vi "ASE_MPC_Experiment_template.vi"() -> ()   [LabVIEW 2018]
uses:
  <vilib>/Simulation/Scripting/Companion Diagram/SimConfigNode/SimParams.ctl
  <vilib>/Simulation/Scripting/Companion Diagram/SimConfigNode/_simSolvers.ctl
  <vilib>/Simulation/Implementation/Shared/SIMSCR Execution Mode.ctl
  <vilib>/Platform/TimedLoop/XDataNode/timing_clust.ctl
  <vilib>/Platform/TimedLoop/XDataNode/nitl_modes.ctl
  <vilib>/Platform/TimedLoop/XDataNode/wakeup.ctl
  <vilib>/Simulation/Param Hierarchy/Typedefs/SIMPH Param Control Actions.ctl
  <vilib>/Simulation/Implementation/Shared/SIM limit type.ctl
  <vilib>/Simulation/Scripting/Editor Utilities/SIM subVI tag data.ctl
  <vilib>/Simulation/Scripting/Editor Utilities/SIM subVI execution type.ctl
  <vilib>/Simulation/Implementation/Shared/NILVSim_ParamChanged.vi
  <vilib>/Simulation/Implementation/Shared/NILVSim_FinishedLate.vi
  <vilib>/Simulation/Implementation/Shared/NILVSIM_BeginStep.vi
  <vilib>/Simulation/Utility/Implementation/SIM Halt.vi
  <vilib>/Simulation/DataSources/Implementation/NILVSim Signal Generator.llb/SIM Signal Generator (scalar).vi
  <vilib>/Simulation/Nonlinear/Implementation/NILVSim Saturation.llb/SIM Saturation (scalar).vi
  <vilib>/Simulation/ContinuousLinear/Implementation/NILVSim Transfer Function.llb/SIM Transfer Function Distributor (SISO).vi
  <vilib>/Simulation/SignalArithmetic/Implementation/NILVSim Gain.llb/SIM Gain (scalar).vi
  <vilib>/Simulation/ContinuousLinear/Implementation/NILVSim Integrator new.llb/SIM Integrator distributor (scalar).vi
  <vilib>/Simulation/ContinuousLinear/Implementation/NILVSim Transfer Function.llb/SIM Transfer Function Collector (SISO).vi
  <vilib>/Simulation/Nonlinear/Implementation/NILVSim RateLimiter.llb/SIM RateLimiter (scalar).vi
  <vilib>/Simulation/Implementation/Shared/SIM Fire Discrete SubVI.vi
  <vilib>/Simulation/ContinuousLinear/Implementation/NILVSim Integrator new.llb/SIM Integrator collector (scalar).vi
  <vilib>/Simulation/Nonlinear/Implementation/NILVSim Saturation.llb/SIM Saturation (vector).vi
  <vilib>/Simulation/SignalArithmetic/Implementation/NILVSim Gain.llb/SIM Gain (vector).vi
  <vilib>/Simulation/Implementation/Shared/NILVSim_Manager.vi
  <vilib>/Utility/error.llb/Clear Errors.vi
  <vilib>/Simulation/Implementation/Shared/NILVSim_FinalizeModel.vi
  <vilib>/Simulation/Implementation/Shared/SIM Fire Discrete SubVI (Core).vi
  <vilib>/imath/engines/lvmath/Plug In/Control Design/BuiltInFunctions/ss/NIMS_CD_ss(A,B,C,D).vi
  <vilib>/imath/engines/lvmath/Plug In/Control Design/BuiltInFunctions/c_to_d/NIMS_CD_c_to_d(SS,TS,STR,DBL).vi
  <vilib>/imath/engines/lvmath2/RunTimeEngine/NodeEndStatement/NIMS_NodeEndStatement_Output.vi
  <instcachedir>/0/NIMS_NodeEndStatement_Output_53EC0D466D134D7ABD903AC30B43404B.lvgen/NIMS_NodeEndStatement_Output_53EC0D466D134D7ABD903AC30B43404B_011.vi
  <vilib>/imath/engines/lvmath2/RunTimeEngine/ErrorHandling/NIMS_Finalize Error.vi
  <vilib>/addons/Control Design/_Model Construction/Model Information.llb/Model Information SubVIs/cd_Get Matrices From SS Model.vi
  <vilib>/imath/engines/lvmath2/RunTimeEngine/IndexRead/NIMS V(R2).vi
  <instcachedir>/0/NIMS V(R2)_C76619605A0E4E9F8B2FA9389712AC47.lvgen/NIMS V(R2)_C76619605A0E4E9F8B2FA9389712AC47_000.vi
  <vilib>/imath/engines/lvmath2/RunTimeEngine/BuiltInFunctions/diag/NIMS_diag.vi
  <instcachedir>/0/NIMS_diag_A176D428AACC4FD18ED77B06CA0A1FE1.lvgen/NIMS_diag_A176D428AACC4FD18ED77B06CA0A1FE1_003.vi
  <vilib>/imathl/engines/lvmath/Functions/Error Handling/Create Error.vi
  <vilib>/imath/engines/lvmath2/RunTimeEngine/IndexRead/NIMS V(S).vi
  <instcachedir>/0/NIMS V(S)_0488751826AF41519A22953C041130DC.lvgen/NIMS V(S)_0488751826AF41519A22953C041130DC_000.vi
  <vilib>/imath/engines/lvmath2/RunTimeEngine/ArithmeticOperatorToken/NIMS_ArithmeticOperator_multmx.vi
  <instcachedir>/0/NIMS_ArithmeticOperator_multmx_622CA76F9646436AB036D42A9A1CE0E6.lvgen/NIMS_ArithmeticOperator_multmx_622CA76F9646436AB036D42A9A1CE0E6_004.vi
  <vilib>/imath/engines/lvmath2/RunTimeEngine/ArithmeticOperatorToken/NIMS_ArithmeticOperator_plus.vi
  <instcachedir>/0/NIMS_ArithmeticOperator_plus_DE670E32103C4C10ADF2A97367172B30.lvgen/NIMS_ArithmeticOperator_plus_DE670E32103C4C10ADF2A97367172B30_003.vi
  <vilib>/imath/engines/lvmath2/RunTimeEngine/ErrorHandling/NIMS_Create Error From Enums.vi
  <vilib>/imath/engines/lvmath2/RunTimeEngine/IndexReplace/NIMS M(S,S)=S.vi
  <instcachedir>/0/NIMS M(S,S)=S_5DAF17B45D8A4C8588C7CF468644990A.lvgen/NIMS M(S,S)=S_5DAF17B45D8A4C8588C7CF468644990A_002.vi
  <vilib>/imath/engines/lvmath2/RunTimeEngine/BuiltInFunctions/eye/NIMS_M=eye(I32, I32).vi
  <vilib>/imath/engines/lvmath2/RunTimeEngine/IndexReplace/NIMS M(R2,$)=M.vi
  <instcachedir>/0/NIMS M(R2,$)=M_E62C22E4B8174738B7B297CD2875EB66.lvgen/NIMS M(R2,$)=M_E62C22E4B8174738B7B297CD2875EB66_002.vi
  <vilib>/imath/engines/lvmath2/RunTimeEngine/RangeToken/NIMS_Range_R2 - Integer.vi
  <instcachedir>/0/NIMS_Range_R2 - Integer_E35B921DECF84AADB7325A02D418BFCC.lvgen/NIMS_Range_R2 - Integer_E35B921DECF84AADB7325A02D418BFCC_001.vi
  <vilib>/imath/engines/lvmath2/RunTimeEngine/CommandStatement/MC_CommandStatement_break.vi
  <vilib>/imath/engines/lvmath2/RunTimeEngine/ArithmeticOperatorToken/NIMS_ArithmeticOperator_powermx(M,M).vi
  <instcachedir>/0/NIMS_ArithmeticOperator_multmx_622CA76F9646436AB036D42A9A1CE0E6.lvgen/NIMS_ArithmeticOperator_multmx_622CA76F9646436AB036D42A9A1CE0E6_006.vi
  <vilib>/imath/engines/lvmath2/RunTimeEngine/MatrixToken/NIMS_MatrixToken_M_M.vi
  <instcachedir>/0/NIMS_MatrixToken_M_M_C5809CB3B49B4BB3BF486E1039DE826B.lvgen/NIMS_MatrixToken_M_M_C5809CB3B49B4BB3BF486E1039DE826B_003.vi
  <instcachedir>/0/NIMS_ArithmeticOperator_multmx_622CA76F9646436AB036D42A9A1CE0E6.lvgen/NIMS_ArithmeticOperator_multmx_622CA76F9646436AB036D42A9A1CE0E6_007.vi
  <vilib>/imath/engines/lvmath2/RunTimeEngine/IndexReplace/NIMS M(R2,R2)=M.vi
  <instcachedir>/0/NIMS M(R2,R2)=M_33171D760B764D5F81A0D4DA8D20878D.lvgen/NIMS M(R2,R2)=M_33171D760B764D5F81A0D4DA8D20878D_000.vi
  <instcachedir>/0/NIMS M(S,S)=S_5DAF17B45D8A4C8588C7CF468644990A.lvgen/NIMS M(S,S)=S_5DAF17B45D8A4C8588C7CF468644990A_000.vi
  <instcachedir>/0/NIMS_ArithmeticOperator_multmx_622CA76F9646436AB036D42A9A1CE0E6.lvgen/NIMS_ArithmeticOperator_multmx_622CA76F9646436AB036D42A9A1CE0E6_003.vi
  <vilib>/imath/engines/lvmath2/RunTimeEngine/RowToken/NIMS_RowToken_M_M.vi
  <instcachedir>/0/NIMS_RowToken_M_M_9381229BAB584C0281F245468A1A9A6C.lvgen/NIMS_RowToken_M_M_9381229BAB584C0281F245468A1A9A6C_003.vi
  <instcachedir>/0/NIMS_ArithmeticOperator_plus_DE670E32103C4C10ADF2A97367172B30.lvgen/NIMS_ArithmeticOperator_plus_DE670E32103C4C10ADF2A97367172B30_011.vi
  <instcachedir>/0/NIMS_NodeEndStatement_Output_53EC0D466D134D7ABD903AC30B43404B.lvgen/NIMS_NodeEndStatement_Output_53EC0D466D134D7ABD903AC30B43404B_002.vi
  <instcachedir>/0/NIMS_NodeEndStatement_Output_53EC0D466D134D7ABD903AC30B43404B.lvgen/NIMS_NodeEndStatement_Output_53EC0D466D134D7ABD903AC30B43404B_003.vi
  <instcachedir>/0/NIMS_NodeEndStatement_Output_53EC0D466D134D7ABD903AC30B43404B.lvgen/NIMS_NodeEndStatement_Output_53EC0D466D134D7ABD903AC30B43404B_012.vi
  <vilib>/FPGAPlugInAG/cRIO-9068/niLvFpga_Open_cRIO-9068.vi
  <vilib>/rvi/interface/common/dynamic/niFpgaDynamicAddResources.vi
  <vilib>/Simulation/Implementation/Shared/SIM Unbundle Sim Info.vi
  <vilib>/Simulation/Implementation/Shared/SIMSH Read Queue.vi
  <vilib>/Simulation/Implementation/Shared/NILVSim_Initialize.vi
  <vilib>/Utility/error.llb/Error Cluster From Error Code.vi
  <vilib>/rvi/errors/niLvFpgaAdjustHostInterfaceError.vi
  <vilib>/Simulation/Utility/Implementation/NILVSim Get Time and IsAcceptedStep.vi
  <vilib>/imath/engines/lvmath2/RunTimeEngine/ArithmeticOperatorToken/NIMS_ArithmeticOperator_multmx(M,CV).vi
  <instcachedir>/0/NIMS_ArithmeticOperator_multmx(M,CV)_2F1CD6A2FE4F4213A4AD1C901C2750F5.lvgen/NIMS_ArithmeticOperator_multmx(M,CV)_2F1CD6A2FE4F4213A4AD1C901C2750F5_002.vi
  <vilib>/imath/engines/lvmath2/RunTimeSupport/NIMS_Complex To Real.vi
  <instcachedir>/0/NIMS_Complex To Real_DC07FF5F56D84FD694198341FF08C5E7.lvgen/NIMS_Complex To Real_DC07FF5F56D84FD694198341FF08C5E7_000.vi
  <vilib>/imath/engines/lvmath2/RunTimeSupport/NIMS_Get Any Vector_w Error - Matrix.vi
  <instcachedir>/0/NIMS_Get Any Vector_w Error - Matrix_1B26302039EC43C7B9FA287B1E12D88C.lvgen/NIMS_Get Any Vector_w Error - Matrix_1B26302039EC43C7B9FA287B1E12D88C_001.vi
  <vilib>/imath/engines/lvmath2/RunTimeEngine/BuiltInFunctions/fmin_qp/NIMS_fmin_qp.vi
  <instcachedir>/0/NIMS_NodeEndStatement_Output_53EC0D466D134D7ABD903AC30B43404B.lvgen/NIMS_NodeEndStatement_Output_53EC0D466D134D7ABD903AC30B43404B_001.vi
  <vilib>/Simulation/Implementation/Shared/NILVSim_GetModelError.vi
  <vilib>/Simulation/Implementation/Shared/SIM Bundle Sim Info.vi
  <vilib>/FPGAPlugInAG/Dynamic/niLvFpga_Close_Dynamic.vi
  <vilib>/Simulation/Scripting/Companion Diagram/SimConfigNode/SimDog.xnode
  <vilib>/rvi/interface/nirviOpenFPGA/nirviOpenFPGA.xnode
  FPGA Bitfiles/MPCASE_FPGATarget_FPGAQ1MODULE_QZL3H99B2Ro.lvbitx
  FPGA_Q1_MODULE.vi
  <vilib>/Quanser/Rapid Control Prototyping Toolkit/discrete/_TypeSpecific/CL Bias Removal (Scalar).vi
  <vilib>/Quanser/Rapid Control Prototyping Toolkit/discrete/CL Bias Removal.vi
  <vilib>/Platform/TimedLoop/XDataNode/XDataNode.xnode
  <vilib>/rvi/interface/nirviReadWriteControl/nirviReadWriteControl.xnode
  <vilib>/Simulation/Implementation/XNodeFramework/SimXNode/SimX.xnode
  <vilib>/rvi/interface/nirviCloseFPGA/nirviCloseFPGA.xnode
  <vilib>/Simulation/ContinuousLinear/Implementation/NILVSim Transfer Function.llb/SIM Transfer Function (SISO).vi
  <vilib>/Simulation/ContinuousLinear/Implementation/NILVSim Integrator new.llb/SIM Integrator (scalar).vi
  <vilib>/rvi/interface/Simulation/niFpgaSimulationCallBeginRW.vi
  <vilib>/addons/Control Design/_Model Construction/NI_LinSys_Model Information.lvlib
  NiFpgaLv.dll
  <vilib>/Platform/TimedLoop/XDataNode/XDNodeRunTimeDep.lvlib
  <vilib>/Simulation/Implementation/Shared/NI_SIM_Implementation.lvlib
panel:
  out "A":dbl[][](array[numeric])
  in  "weight O4":dbl
  in  "weight O3":dbl
  in  "weight I1":dbl
  in  "weight O2":dbl
  in  "weight O1":dbl
  in  "Control Horizon (Nc)":u64 step=1
  in  "Prediction Horizon (Np)":u64 step=1
  in  "Enable motor":bool
  in  "Setpoint Command 2":T1={"Amplitude (m)"=0.01, "Frequency (Hz)"=0.3} caption="Road (Bottom Plate)\nAmplitude Command (m)" {"Frequency (Hz)" min=0.0 max=0.5 step=0.009999999776482582 format="%_3f"; "Amplitude (m)" min=-10.0 max=10.0 step=0.5 format="%_3f"}
  out "Active Suspension Motor Voltage (V)":dbl(graph)
  in  "Enable active suspension":bool
  out "Zr(m), Zs(m), Zus(m) 2":T2(graph)={"output"=0.0096065956, "Result"=0.0090666584, "output"=0.0091514816}
  out "Accelerometer Signal":dbl(graph)
  in  "Halt?":bool
  # "Active Suspension MPC"
  # "MPC parameters"
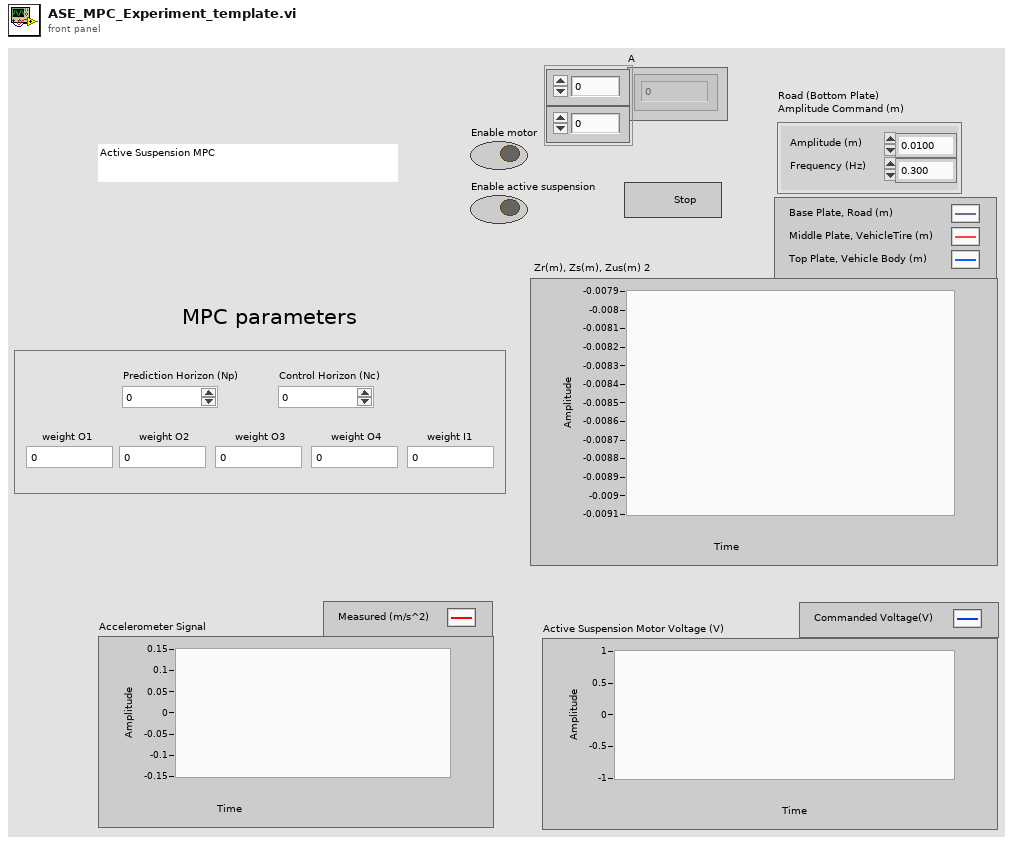
[diagram p1: front panel]
types:
  T1 = cluster{"Amplitude (m)":dbl, "Frequency (Hz)":dbl}
  T2 = cluster{"output":dbl, "Result":dbl, "output":dbl}
  T3 = typedef "SIMSCR Execution Mode.ctl" = enum16{"Simulate to Completion", "Single Time-Step Simulation (Fixed Step Only)"}
  T4 = typedef "XDNodeRunTimeDep.lvlib/timing_clust.ctl" = cluster{"Expected End [f-1]":u64, "Actual End [f-1]":u64, "Finished Late? [f-1]":bool, "Expected End [i-1]":u64, "Actual End [i-1]":u64, "Finished Late? [i-1]":bool, "Expected Start [i]":u64, "Actual Start [i]":u64, "Expected Start [f]":u64, "Actual Start [f]":u64, "Source Name":string, "Structure Name":string, "Period":i64, "Deadline":i64, "Offset":i64, "Start":i64, "Priority":i32, "Timeout":i32, "Mode":T5, "Wakeup Reason":T6, "Error":errorcluster, "Source Type":string, "Secondary Source Type":string, "Global End Time":u64, "Global Start Time":u64, "Frame Duration":u64, "Iteration Duration":u64, "Assigned CPU":i32, "I/O Scan Engine Mode":u32}
  T5 = typedef "XDNodeRunTimeDep.lvlib/nitl_modes.ctl" = enum32{"No Change", "Process missed periods, maintain original phase", "Discard missed periods, maintain original phase", "Process missed periods, ignore original phase", "Discard missed periods, ignore original phase"}
  T6 = typedef "XDNodeRunTimeDep.lvlib/wakeup.ctl" = enum32{"Normal", "Aborted", "Asynchronous wakeup", "Timing source error", "Timed loop error", "Timeout"}
  T7 = typedef "SIMPH Param Control Actions.ctl" = enum16{"get params", "set params"}
  T8 = typedef "SIM subVI tag data.ctl" = cluster{"period":dbl, "skew":dbl, "Simulation execution type":T9}
  T9 = typedef "SIM subVI execution type.ctl" = enum16{"Function call", "Discrete", "Continuous", "Initialization only", "Final step only"}
  T10 = typedef "SIM limit type.ctl" = enum16{"upper", "lower", "both", "none"}
  T11 = cluster{"SIMSH Sim Time":dbl, "CL Enabled Moving Average (Scalar)":cluster{"output":dbl}, "CL Enabled Moving Average (Scalar) - SIMSH":cluster{"SIMSH Sim Time":dbl, "Memory 2":cluster{"output":dbl[]}, "states on enable":enum16{"reset average", "cumulative average"}, "Select 2":cluster{"s? t:f":dbl}, "Memory":cluster{"output":dbl}, "Index Array 2":cluster{"element":dbl}, "Divide 2":cluster{"x/y":dbl}, "Select":cluster{"s? t:f":dbl[]}, "Summation":cluster{"Result":dbl[]}, "Discrete Delay":cluster{"output":dbl[]}, "Not":cluster{".not. x?":bool}, "Initialize Array 3":cluster{"initialized array":dbl[]}, "Array Size 2":cluster{"size(s)":i32}, "Build Array":cluster{"appended array":dbl[]}}, "initial value":dbl, "Select":cluster{"s? t:f":dbl}, "Not":cluster{".not. x?":bool}, "Subtract":cluster{"x-y":dbl}, "And":cluster{"x .and. y?":bool}, "Less?":cluster{"x < y?":bool}, "Greater Or Equal?":cluster{"x >= y?":bool}, "Simulation Time":cluster{"simulation time":dbl}}
  T12 = typedef "SimParams.ctl" = cluster{"Initial Time (s)":dbl, "Final Time (s)":dbl, "Step Size (s)":dbl, "ODE Solver":T13, "Minimum Step Size (s)":dbl, "Maximum Step Size (s)":dbl, "Relative Tolerance":dbl, "Absolute Tolerance":dbl, "Software Timing":bool, "Initial Step Size (s)":dbl, "Automatic Fixed Step Size?":bool, "Automatic Discrete Step Size?":bool, "Discrete Step Size (s)":dbl, "Calculate using Time Step":bool, "Solver Wired?":bool, "Prev.Frm.Expected End":u64, "Prev.Frm.Actual End":u64, "Prev.Frm.Finished Late?":bool, "Prev.Iter.Expected End":u64, "Prev.Iter.Actual End":u64, "Prev.Iter.Finished Late?":bool, "Expected Iteration Start":u64, "Actual Iteration Start":u64, "Expected Frame Start":u64, "Actual Frame Start":u64, "Source Name":string, "Name":string, "Period":i64, "Deadline":i64, "Offset":i64, "Start":i64, "Priority":i32, "Timeout":i32, "Processor":i32, "Mode":enum32{"No Change", "Process missed periods, maintain original phase", "Discard missed periods, maintain original phase", "Process missed periods, ignore original phase", "Discard missed periods, ignore original phase"}, "Wakeup reason":enum32{"Normal", "Aborted", "Asynchronous wakeup", "Timing source error", "Timed loop error", "Timeout"}, "Error":errorcluster, "Source Type":string, "Secondary Source Type":string, "Global End Time":u64, "Global Start Time":u64, "Full Solver Reset":bool, "Execution Mode":T3, "Nan/Inf Check":bool, "Custom Solver Library":string, "Solver Is Variable":bool, "custom solver name":string, "Signal Collection Decimation":u32}
  T13 = typedef "_simSolvers.ctl" = enum16{"Runge-Kutta 1 (Euler)", "Runge-Kutta 2", "Runge-Kutta 3", "Runge-Kutta 4", "Runge-Kutta 23 (variable)", "Runge-Kutta 45 (variable)", "BDF (variable)", "Adams-Moulton (variable)", "Rosenbrock (variable)", "Discrete States Only", "SDIRK 4 (variable)", "Radau 5 (variable)", "Radau 9 (variable)", "Radau 13 (variable)", "Radau [Variable Order] (variable)", "Gear's Method (variable)", "Linearizer", "State Query", "Trim Eval", "Custom Solver"}
  T14 = typedef "NI_LinSys_Model Typedefs.lvlib/CD State Space Model (MIMO).ctl" = cluster{"properties":T15, "A":dbl[][], "B":dbl[][], "C":dbl[][], "D":dbl[][], "StateNames":string[], "Transport Delay":dbl[][]}
  T15 = typedef "NI_LinSys_Model Typedefs.lvlib/CD General Elements.ctl" = cluster{"Model name":string, "Input names":string[], "Output names":string[], "Input Delays":dbl[], "Output Delays":dbl[], "Sampling Time":dbl, "Notes":string}
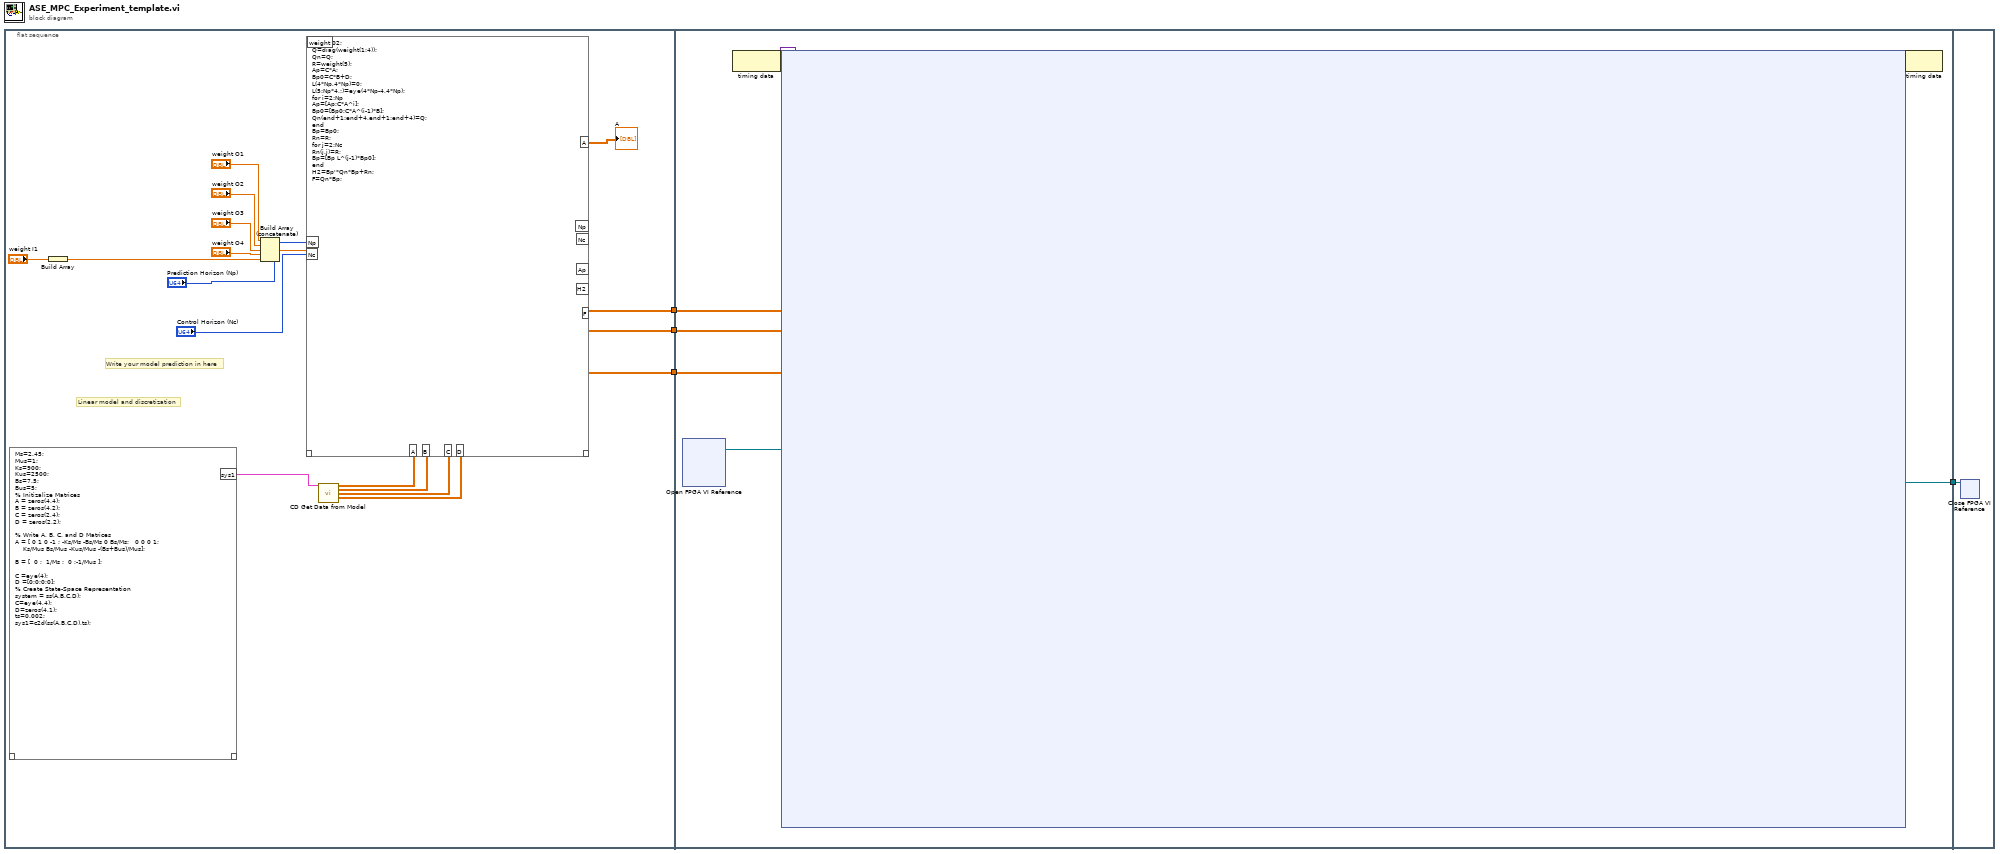
[diagram p0: block diagram]
diagram:
  n1 = flat-sequence {
    tunnel: [w15] -> w3
    tunnel: [w14] -> w2
    tunnel: [w13] -> w1
    tunnel: [w759] -> w4
    tunnel: w3 -> [w758]
    tunnel: w2 -> [w757]
    tunnel: w1 -> [w756]
    tunnel: w4 -> [w1951]
    frame #0 {
      # "Write your model prediction in here"
      # "Linear model and discretization"
      n2 = mathscript code="Ms=2.45;\nMus=1;\nKs=900;\nKus=2500;\nBs=7.5;\nBus=5;\n% Initizalize Matrices\nA = zeros(4,4);\nB = zeros(4,2);\nC = zeros(2,4);\nD = zeros(2,2);\n\n% Write A, B, C, and D Matrices\nA = [ 0 1 0 -1 ; -Ks/Ms -Bs/Ms 0 Bs/Ms;   0 0 0 1;\n    Ks/Mus Bs/Mus -Kus/Mus -(Bs+Bus)/Mus];\n\nB = [  0 ;  1/Ms ;  0 ;-1/Mus ];\n\nC =eye(4);\nD =[0;0;0;0];\n% Create State-Space Representation\nsystem = ss(A,B,C,D);\nC=eye(4,4);\nD=zeros(4,1);\nts=0.002;\nsys1=c2d(ss(A,B,C,D),ts);"() -> ("sys1"=w12:T14)  [unwired: 1 in, 1 out]
      n3 = Build Array ("Build Array 4")("weight I1") -> (w17:dbl[])
      n4 = Build Array (concatenate) ("Build Array 3")("weight O1", "weight O2", "weight O3", "weight O4", w17) -> (w16:dbl[])
      n5 = call-poly <vilib>:"CD Get Data from Model.vi"("State-Space Model"=w12) -> ("Matrix A"=w11:dbl[][], "Matrix B"=w9:dbl[][], "Matrix C"=w10:dbl[][], "Matrix D"=w8:dbl[][])  [unwired: 10 in, 1 out]
      n6 = mathscript code="ts=0.002;\nQ=diag(weight(1:4));\nQn=Q;\nR=weight(5);\nAp=C*A;\nBp0=C*B+D;\nL(4*Np,4*Np)=0;\nL(5:Np*4,:)=eye(4*Np-4,4*Np);\nfor i=2:Np\nAp=[Ap;C*A^i];\nBp0=[Bp0;C*A^(i-1)*B];\nQn(end+1:end+4,end+1:end+4)=Q;\nend\nBp=Bp0;\nRn=R;\nfor j=2:Nc\nRn(j,j)=R;\nBp=[Bp L^(j-1)*Bp0];\nend\nH2=Bp'*Qn*Bp+Rn;\nF=Qn*Bp;" ("MathScript Node 2")("Np"="Prediction Horizon (Np)", "Nc"="Control Horizon (Nc)", "weight"=w16, "A"=w11, "B"=w9, "C"=w10, "D"=w8) -> ("Ap"=w15:cdb[][], "F"=w13:cdb[][], "H2"=w14:cdb[][], "A"=→"A":dbl[][])  [unwired: 1 in, 3 out]
    }
    frame #1 {
      n7 = xnode "Open FPGA VI Reference"() -> ("FPGA VI Reference Out"=w760:refnum<k20>)  [unwired: 2 in, 1 out]
      n8 = node-c288() -> (w762:variant)  [unwired: 1 in]
      n9 = node-c254 ("Control & Simulation Loop")(w762, w760, w758, w757, w756) -> (w761:variant, w759:refnum<k20>)
      n10 = node-c288(w761) -> ()  [unwired: 1 out]
    }
    frame #2 {
      n11 = xnode "Close FPGA VI Reference"("FPGA VI Reference In"=w1951) -> ()  [unwired: 1 in, 1 out]
    }
  }
